vi "Initial_queues.vi"() -> (0 "Queues":T1)   [LabVIEW 2015]
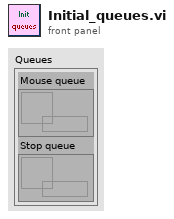
[diagram p1: front panel]
types:
  T1 = cluster{"Mouse queue":refnum<queue>, "Stop queue":refnum<queue>}
  T2 = cluster{"device ID":refnum<k1>, "axis info":cluster{"Horizontal":i32, "Vertical":i32, "Scrolling":i32}, "button info":cluster{"button 1":bool, "button 2":bool, "button 3":bool, "button 4":bool}}
  T3 = cluster{"queue out":refnum<queue>, "queue out":refnum<queue>}
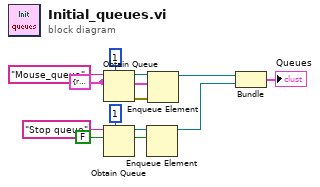
[diagram p0: block diagram]
diagram:
  w4 = FALSE
  w8 = T2 {"device ID"=refnum, "axis info"={"Horizontal"=0, "Vertical"=0, "Scrolling"=0}, "button info"={"button 1"=FALSE, "button 2"=FALSE, "button 3"=FALSE, "button 4"=FALSE}}
  n1 = Obtain Queue(max queue size (-1, unlimited)=1, name (unnamed)="Mouse_queue", element data type=w8) -> (queue out=w9:refnum<queue>, error out=w10:errorcluster)  [unwired: 2 in, 1 out]
  n2 = Obtain Queue(max queue size (-1, unlimited)=1, name (unnamed)="Stop queue", element data type=w4) -> (queue out=w6:refnum<queue>)  [unwired: 2 in, 2 out]
  n3 = Enqueue Element(queue=w6, element=w4) -> (queue out=w2:refnum<queue>)  [unwired: 2 in, 2 out]
  n4 = Enqueue Element(queue=w9, element=w8, error in (no error)=w10) -> (queue out=w3:refnum<queue>)  [unwired: 1 in, 2 out]
  n5 = Bundle("queue out"=w3, "queue out"=w2) -> (→"Queues":T3)  [unwired: 1 in]
